vi "WayPointCheckoff.vi"() -> ()   [LabVIEW 2012]
uses:
  3-2--pre-class-branch/Software/0x2-OCU-Think Comm/0x2 Typedefs/waypointTypes.ctl
  3-2--pre-class-branch/Software/2-Think/2 Typedefs/UTM Location.ctl
  3-2--pre-class-branch/Software/0x2-OCU-Think Comm/0x2 Typedefs/ocuWaypoint.ctl
  3-2--pre-class-branch/Software/0x2-OCU-Think Comm/0x2 Typedefs/Waypoints List.ctl
panel:
  in  "Timeout\nCancellation\nBuffer":dbl
  in  "Timeout Buffer":dbl
  in  "Timeout Time":dbl
  in  "Checkoff Buffer":dbl
  out "Checked Off?":bool=TRUE
  out "Timed Out?":bool=TRUE
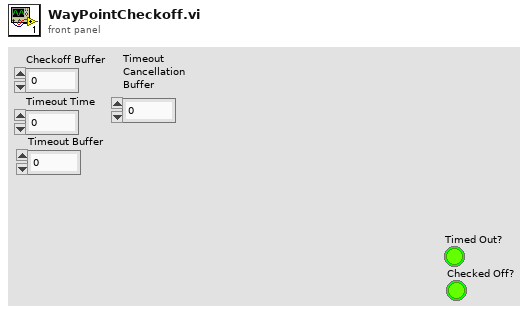
[diagram p1: front panel]
types:
  T1 = typedef "Waypoints List.ctl" = T2[]
  T2 = typedef "ocuWaypoint.ctl" = cluster{"Point Type":T3, "Dist/Time":dbl, "UTM Location":T4}
  T3 = typedef "waypointTypes.ctl" = enum16{"Drive", "Round Port", "Round Starboard", "Stay"}
  T4 = typedef "UTM Location.ctl" = cluster{"UTM Zone":dbl, "Hemisphere":enum16{"North", "South"}, "East":dbl, "North":dbl}
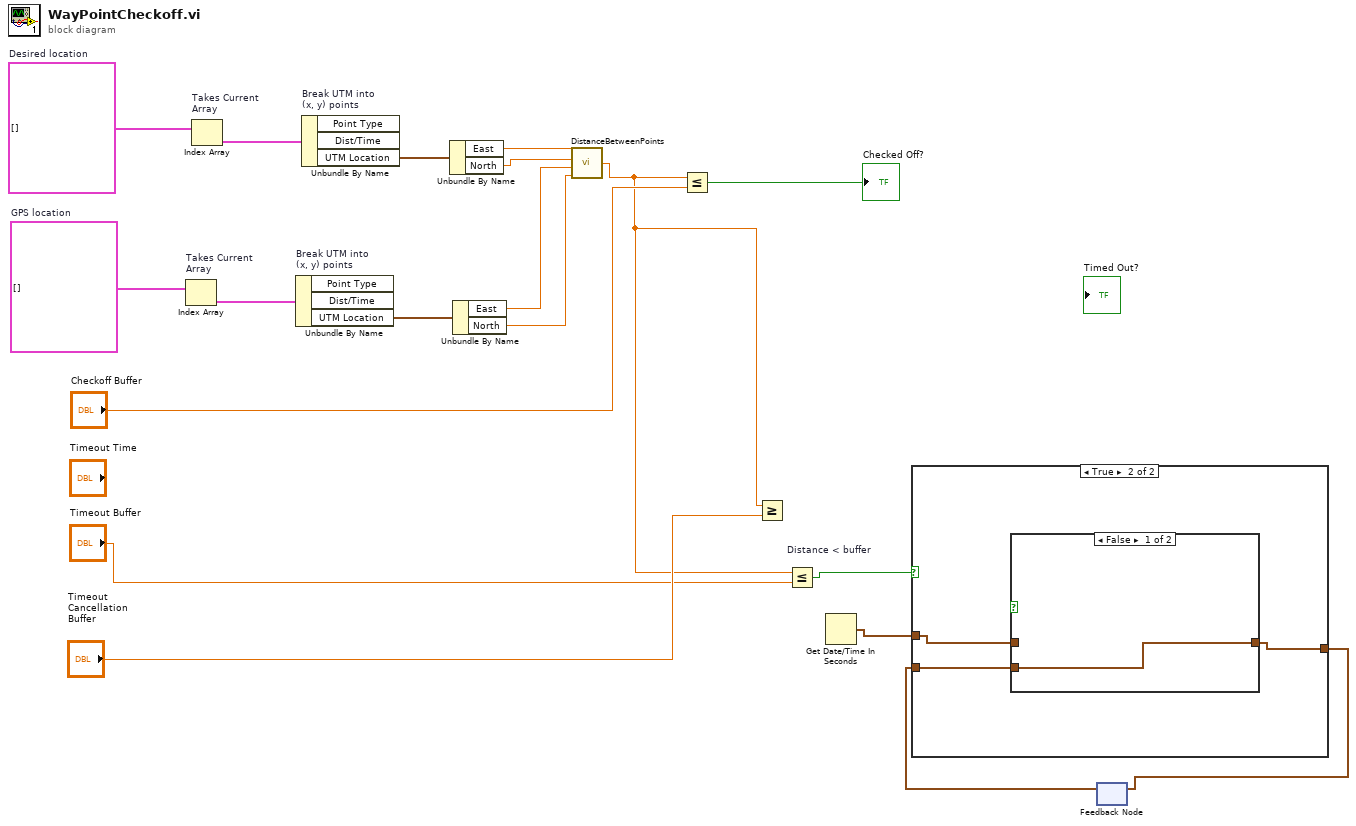
[diagram p0: block diagram]
diagram:
  w19 = T1 []  # Desired location
  w14 = T1 []  # GPS location
  n1 = Index Array "Takes Current\nArray"(array=w14) -> (element=w16:T2)  [unwired: 1 in]
  n2 = Index Array "Takes Current\nArray"(array=w19) -> (element=w18:T2)  [unwired: 1 in]
  n3 = Unbundle By Name "Break UTM into\n(x, y) points"(w16) -> ("UTM Location"=w15:T4)  [unwired: 2 out]
  n4 = Unbundle By Name "Break UTM into\n(x, y) points"(w18) -> ("UTM Location"=w17:T4)  [unwired: 2 out]
  n5 = Unbundle By Name(w17) -> ("East"=w13:dbl, "North"=w12:dbl)
  n6 = Unbundle By Name(w15) -> ("East"=w11:dbl, "North"=w10:dbl)
  n7 = call "DistanceBetweenPoints.vi"("coordinate 2\nnorth"=w10, "coordinate 2\neast"=w11, "coordinate 1\nnorth"=w12, "coordinate 1\neast"=w13) -> ("Numeric"=w6:dbl)
  n8 = Less Or Equal?(x=w6, y="Checkoff Buffer") -> (x <= y?=→"Checked Off?":bool)
  n9 = Greater Or Equal? ("distance > buffer")(x=w6, y="Timeout\nCancellation\nBuffer") -> ()  [unwired: 1 out]
  n10 = Less Or Equal? "Distance < buffer"(x=w6, y="Timeout Buffer") -> (x <= y?=w4:bool)
  n11 = Get Date/Time In Seconds() -> (seconds since 1Jan1904=w3:timestamp)
  n12 = feedback #1() -> (w1:timestamp)  [unwired: 1 in]
  n13 = case shown="True" w4 {
    tunnel: w3 -> [_ w21]
    tunnel: [_ w22] -> w2
    tunnel: w1 -> [_ w20]
    frame False {
    }
    frame True {
      n14 = case shown="False" {
        selector: _ -> [_ _]
        tunnel: w21 -> [_ w24]
        tunnel: [w23 w24] -> w22
        tunnel: w20 -> [w23 _]
        frame False {
        }
        frame True {
        }
      }
    }
  }
  n15 = feedback-in #1(w2) -> ()
